vi "Read Renderer.vi"(8 "Error In":errorcluster, 11 "Compiler In":refnum<class "Compiler.lvclass">) -> (0 "Error Out":errorcluster, 2 "Renderer":refnum<class "Renderer.lvclass">, 3 "Compiler Out":refnum<class "Compiler.lvclass">)   [LabVIEW 2018, in "Toolkit.lvlib" / "Compiler.lvclass"]
uses:
  Compiler.lvclass
  Renderer/Renderer.lvclass
  Compiler.lvclass/Compiler.ctl
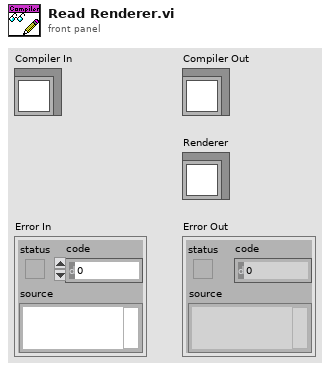
[diagram p1: front panel]
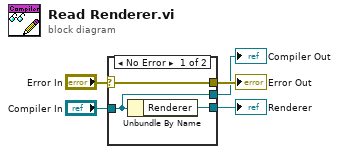
[diagram p0: block diagram]
diagram:
  n1 = case shown="No Error" "Error In" {
    selector: "Error In" -> [w8 w9]
    tunnel: [w8 w9] -> w4
    tunnel: [w7 w10] -> w2
    tunnel: "Compiler In" -> [w7 w10]
    tunnel: [w6 _] -> w1
    frame No Error {
      n2 = Unbundle By Name(w7) -> ("Renderer"=w6:refnum<class "Renderer.lvclass">)
    }
    frame Error {
    }
  }
  "Error Out" <- w4
  "Compiler Out" <- w2
  "Renderer" <- w1
